vi "Dequeue Msg.vi"(8 "error in (no error)":errorcluster, 11 "Queue in":refnum<queue>) -> (0 "error out":errorcluster, 1 "Message":string, 2 "Data":variant, 3 "Queue out":refnum<queue>)   [LabVIEW 2020]
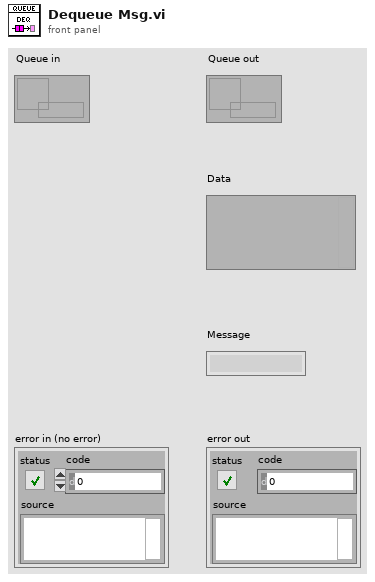
[diagram p1: front panel]
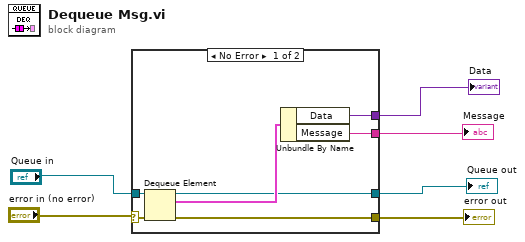
[diagram p0: block diagram]
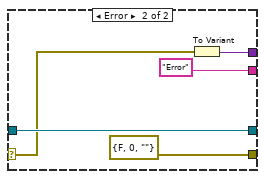
[diagram p2: hidden frame]
diagram:
  n1 = case shown="No Error" "error in (no error)" {
    selector: "error in (no error)" -> [w13 w15]
    tunnel: "Queue in" -> [w12 w18]
    tunnel: [w10 w18] -> w3
    tunnel: [w9 errorcluster {"status"=FALSE, "code"=0, "source"=""} ("error out")] -> w4
    tunnel: [w8 "Error" ("Message")] -> w5
    tunnel: [w7 w16] -> w6
    frame No Error {
      n2 = Dequeue Element(queue=w12, error in (no error)=w13) -> (queue out=w10:refnum<queue>, element=w11:cluster{"Message":string, "Data":variant}, error out=w9:errorcluster)  [unwired: 1 in, 1 out]
      n3 = Unbundle By Name(w11) -> ("Data"=w7:variant, "Message"=w8:string)
    }
    frame Error {
      n4 = To Variant(anything=w15) -> (Variant=w16:variant)
    }
  }
  "Data" <- w6
  "Message" <- w5
  "error out" <- w4
  "Queue out" <- w3
